vi "Add Dummy Grand Children.vi"(8 "error in (no error)":errorcluster, 9 "Folder Names":refnum<class "UTF-8 String.lvclass">[](array[class]), 10 "Parent Tag":refnum<class "UTF-8 String.lvclass">, 11 "Tree In":refnum<vi>) -> (0 "error out":errorcluster, 1 "Folder Names Dup":refnum<class "UTF-8 String.lvclass">[](array[class]), 2 "Parent Tag Dup":refnum<class "UTF-8 String.lvclass">, 3 "Tree Out":refnum<vi>)   [LabVIEW 2020, in "Tree Browser.lvlib"]
doc: "Adds a placeholder grandchild under each child of the parent node where the child directory listing contains folders. This means the tree can display the expand/contract symbol.\n\nNote that all the grandchildren aren't added to the tree here (ie. the full directory listing of a child) because it is simply too slow to build the tree this way (for example navigating to C:\\Windows which is roughly 20k nested folders will make LabVIEW crawl)."
uses:
  Tree Browser.lvlib
  Types/UTF-8 String/UTF-8 String.lvclass
  Types/UTF-8 String/UTF-8 String.lvclass/UTF-8 String.ctl
  Types/UTF-8 Path/UTF-8 Path.lvclass/UTF-8 Path.ctl
  960df1fc-78e5-4513-97f3-4bcba7509537.vi
  1236fc90-e4af-472f-9a2f-7c4441289523.vi
  e390b052-22e5-412d-b29f-a61e40a6b25e.vi
  40a0563b-1fa9-4692-9a2c-eca7a1834d6a.vi
  77a72e39-bbed-4f78-9efc-f095f2d7a7a7.vi
  Private/Conversion/Text as Encoded Path.vi
  Private/Conversion/Polymorphic VIs/Text as Encoded Path (UTF-8 String).vi
  Types/UTF-8 Path/Write Encoded UTF-8 Path.vi
  Types/UTF-8 String/Write Encoded UTF-8 String.vi
  Private/Conversion/Path as UTF-8 Path.vi
  Private/Conversion/Polymorphic VIs/Path as UTF-8 Path (UTF-8 Path).vi
  1236fc90-e4af-472f-9a2f-7c4441289523.vi/5269e09c-4216-478e-8686-9fb7d38e224a.vi
  1236fc90-e4af-472f-9a2f-7c4441289523.vi/d1f4a45d-6f02-44dd-a40b-2b28d80e6519.vi
  Private/Conversion/String as Encoded String.vi
  Private/Conversion/Polymorphic VIs/String as Encoded String (UTF-8 String).vi
  Private/Library/gu_list_folder.vi
  1236fc90-e4af-472f-9a2f-7c4441289523.vi/8eb4f0ed-0012-4550-978e-be3f7301df70.vi
  1236fc90-e4af-472f-9a2f-7c4441289523.vi/f7e6584c-01ed-423f-9bcd-660954191d0d.vi
  Private/Conversion/Polymorphic VIs/Text as Encoded Path (LabVIEW String).vi
  Private/Conversion/Path as Encoded Path.vi
  Private/Conversion/Polymorphic VIs/Path as Encoded Path (UTF-8 Path).vi
  Private/Conversion/Text as Encoded String.vi
  Private/Conversion/Polymorphic VIs/Text as Encoded String (UTF-8 Path).vi
  1236fc90-e4af-472f-9a2f-7c4441289523.vi/5269e09c-4216-478e-8686-9fb7d38e224a.vi/c24c063b-f849-48a1-b323-238a063d7118.vi
  1236fc90-e4af-472f-9a2f-7c4441289523.vi/5269e09c-4216-478e-8686-9fb7d38e224a.vi/a2fd6c11-d594-45c9-8624-1f0a1df69df3.vi
  1236fc90-e4af-472f-9a2f-7c4441289523.vi/5269e09c-4216-478e-8686-9fb7d38e224a.vi/1fd3173e-d32e-42cb-8f0d-819132eb8e27.vi
  1236fc90-e4af-472f-9a2f-7c4441289523.vi/5269e09c-4216-478e-8686-9fb7d38e224a.vi/bb7c39fc-ad8e-447d-bc50-468674bfb562.vi
  Private/Library/Result To Error.vi
  1236fc90-e4af-472f-9a2f-7c4441289523.vi/8eb4f0ed-0012-4550-978e-be3f7301df70.vi/3a31b270-3bb6-4c58-a256-c5fcc2c98f09.vi
  1236fc90-e4af-472f-9a2f-7c4441289523.vi/8eb4f0ed-0012-4550-978e-be3f7301df70.vi/0ec5df2d-ef9b-4f84-a6a8-ffcedd45c4dc.vi
  Private/Conversion/Text as String.vi
  Private/Conversion/Polymorphic VIs/Text as String (UTF-8 Path).vi
  Private/Conversion/Text to UTF-8.vi
  Private/Conversion/Polymorphic VIs/Text to UTF-8 (LabVIEW String).vi
  Types/UTF-8 Path/Read Encoded UTF-8 Path.vi
  Private/Library/gu_string_subset.vi
  Private/Library/gu_to_lower_case.vi
  Private/Library/gu_search_split_string.vi
  Private/Conversion/Polymorphic VIs/String as Encoded String (LabVIEW String).vi
  Private/Conversion/Polymorphic VIs/Text as Encoded String (UTF-8 String).vi
  Private/Conversion/Polymorphic VIs/Text as Encoded String (LabVIEW String).vi
  Private/Memory/Copy String.vi
  Private/Memory/Copy String.vi/4d47babd-4a2d-4eb7-b91b-7e707d692665.vi
  Private/Library/gu_free.vi
  <vilib>/Utility/error.llb/Error Cluster From Error Code.vi
  Private/Memory/Copy String Array.vi
  File IO/Path to Short Name (Unicode).vi
  Types/UTF-8 Path/UTF-8 Path.lvclass
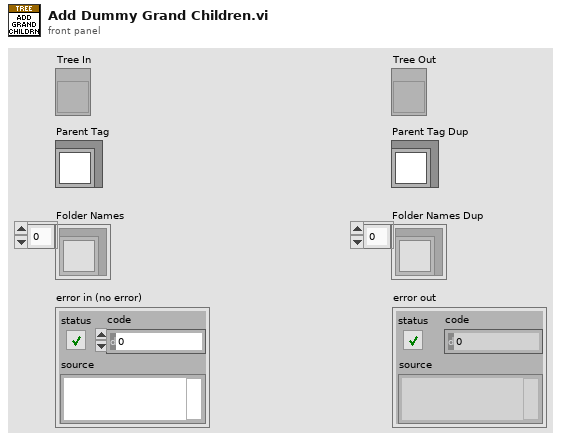
[diagram p1: front panel]
types:
  T1 = typedef "G-Unicode.lvlib/Encoded UTF-8 String.ctl" = string
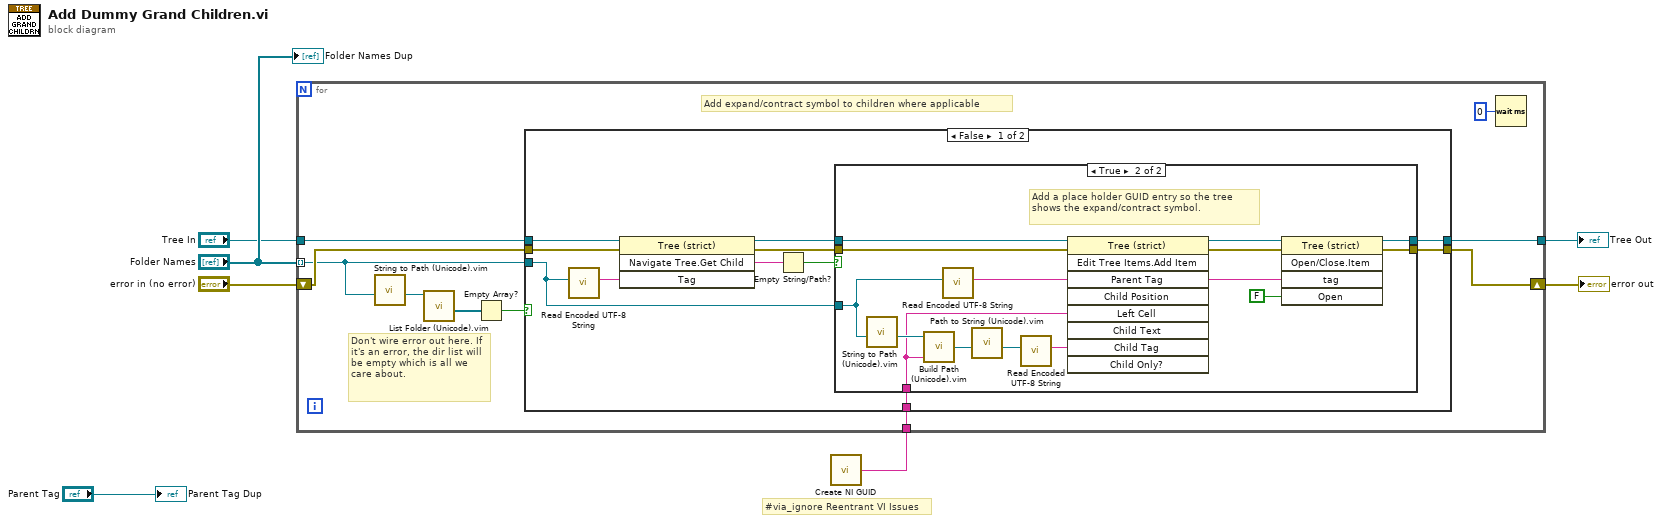
[diagram p0: block diagram]
diagram:
  # "#via_ignore Reentrant VI Issues"
  n1 = call <vilib>:"Create NI GUID.vi"() -> ("NI GUID"=w1:string)
  n2 = for {
    tunnel: "Tree In" -> [w16]
    tunnel: "Folder Names" -> [w8] mode=indexing
    tunnel: w1 -> [w15]
    tunnel: [w14] -> w4
    shift-right: [w12] -> w2
    shift-left: "error in (no error)" -> [w13]
    # "Don't wire error out here. If it's an error, the dir list will be empty which is all we care about."
    # "Add expand/contract symbol to children where applicable"
    n3 = call "String to Path (Unicode).vim"("String"=w8) -> ("Path"=w10:refnum<class "UTF-8 Path.lvclass">)  [unwired: 9 in, 1 out]
    n4 = call "List Folder (Unicode).vim"("Path"=w10) -> ("Folder Names"=w11:refnum<class "UTF-8 String.lvclass">[])  [unwired: 7 in, 3 out]
    n5 = Empty Array?(array=w11) -> (empty?=w17:bool)
    n6 = case shown="False" w17 {
      tunnel: w16 -> [w27 w46]
      tunnel: w8 -> [w24 _]
      tunnel: w15 -> [w23 _]
      tunnel: [w22 w46] -> w14
      tunnel: w13 -> [w21 w45]
      tunnel: [w19 w45] -> w12
      frame False {
        n7 = call "Read Encoded UTF-8 String.vi"("UTF-8 String"=w24) -> ("Encoded UTF-8 String"=w18:T1)  [unwired: 10 in]
        n8 = invoke class="Tree (strict)" method="Navigate Tree.Get Child"(reference=w27, error in=w21, "Tag"=w18) -> (reference out=w25:refnum<vi>, error out=w20:errorcluster, "Navigate Tree:Get Child"=w28:string)  [unwired: 1 in, 1 out]
        n9 = Empty String/Path?(string/path=w28) -> (empty?=w26:bool)
        n10 = case shown="True" w26 {
          tunnel: w25 -> [w30 w44]
          tunnel: w24 -> [_ w34]
          tunnel: w23 -> [_ w42]
          tunnel: [w30 w39] -> w22
          tunnel: w20 -> [w29 w38]
          tunnel: [w29 w36] -> w19
          frame False {
            # "The node already has children."
          }
          frame True {
            # "Add a place holder GUID entry so the tree shows the expand/contract symbol."
            n11 = call "String to Path (Unicode).vim"("String"=w34) -> ("Path"=w43:refnum<class "UTF-8 Path.lvclass">)  [unwired: 9 in, 1 out]
            n12 = call "Build Path (Unicode).vim"("Base Path"=w43, "Name or Relative Path"=w42) -> ("Appended Path"=w33:refnum<class "UTF-8 Path.lvclass">)  [unwired: 6 in, 1 out]
            n13 = call "Read Encoded UTF-8 String.vi"("UTF-8 String"=w34) -> ("Encoded UTF-8 String"=w35:T1)  [unwired: 10 in]
            n14 = call "Path to String (Unicode).vim"("Path"=w33) -> ("String"=w32:refnum<class "UTF-8 String.lvclass">)  [unwired: 9 in, 1 out]
            n15 = call "Read Encoded UTF-8 String.vi"("UTF-8 String"=w32) -> ("Encoded UTF-8 String"=w31:T1)  [unwired: 10 in]
            n16 = invoke class="Tree (strict)" method="Edit Tree Items.Add Item"(reference=w44, error in=w38, "Parent Tag"=w35, "Left Cell"=w42, "Child Tag"=w31) -> (reference out=w41:refnum<vi>, error out=w37:errorcluster)  [unwired: 4 in, 7 out]
            n17 = invoke class="Tree (strict)" method="Open/Close.Item"(reference=w41, error in=w37, "tag"=w35, "Open"=FALSE ("Open?")) -> (reference out=w39:refnum<vi>, error out=w36:errorcluster)  [unwired: 1 in, 3 out]
          }
        }
      }
      frame True {
      }
    }
    n18 = Wait (ms)(milliseconds to wait=u32 0) -> ()  [unwired: 1 out]
  }
  "Tree Out" <- w4
  "error out" <- w2
  "Parent Tag Dup" <- "Parent Tag"
  "Folder Names Dup" <- "Folder Names"
